vi "L1_selectFile.vi"(7 "Function":T1(ring), 9 "File_Name":string[](array[string]), 11 "dup path":path) -> (1 "FileName":string[](array[string]), 3 "FileName_path":path[](array[path]))   [LabVIEW 2023]
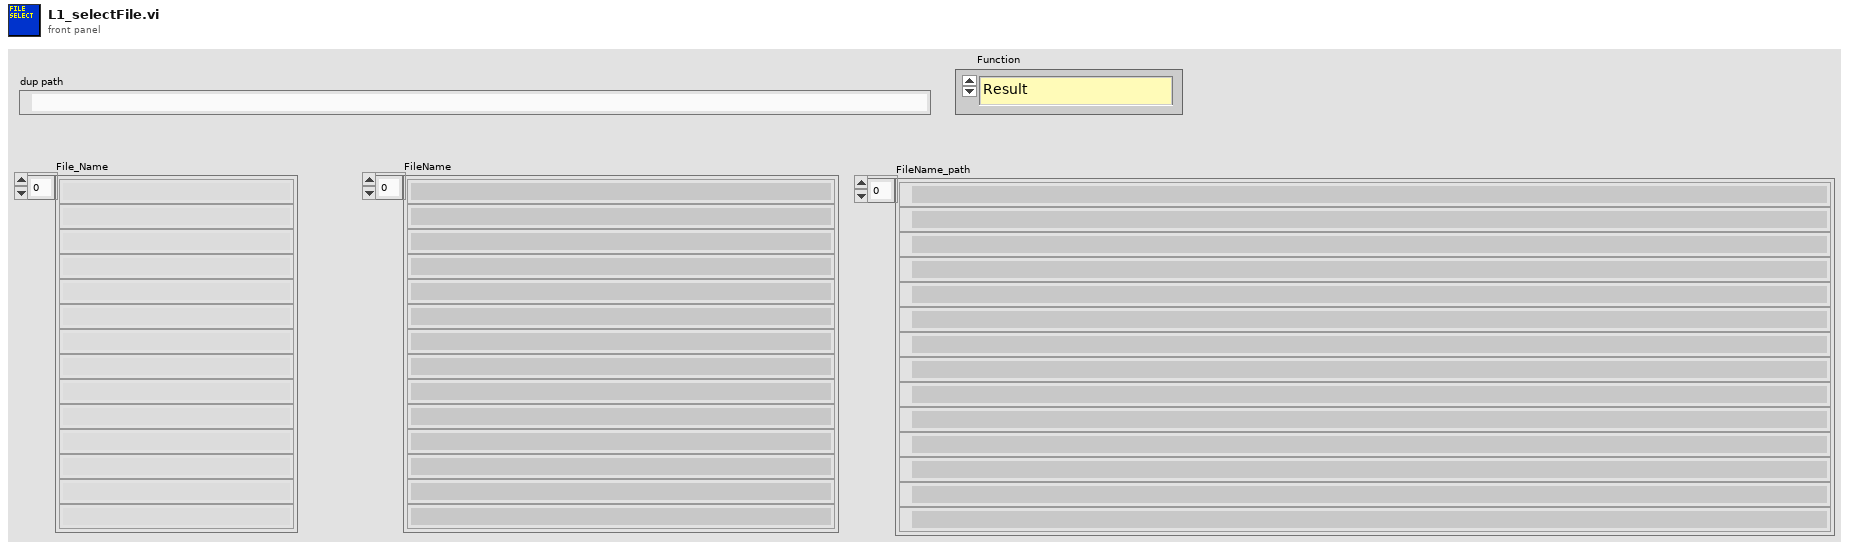
[diagram p1: front panel]
types:
  T1 = enum16{"Result", "Marker_1_26.5GHz", "Marker_2_28GHz", "Marker_3_29.5GHz", "Marker_4_31GHz"}
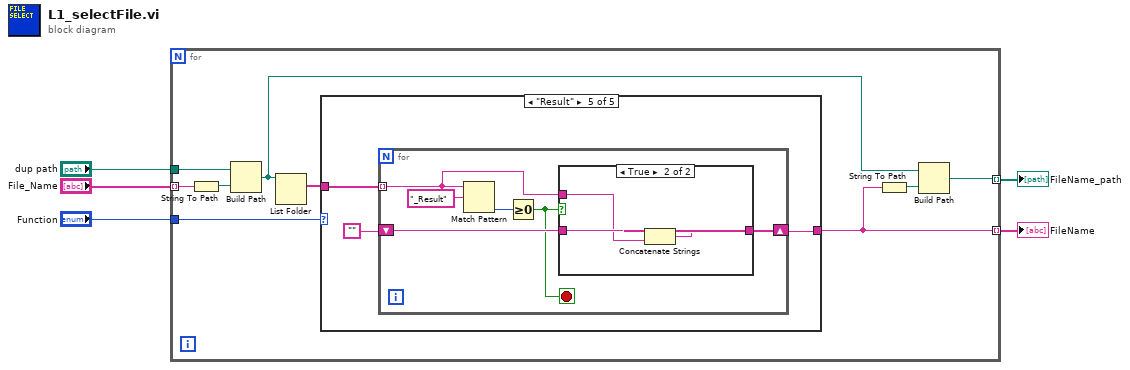
[diagram p0: block diagram]
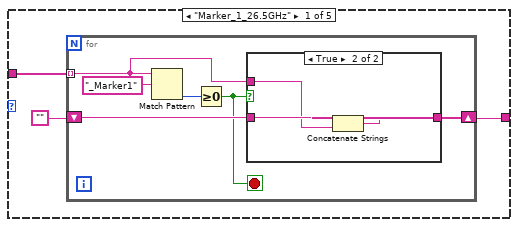
[diagram p2: hidden frame]
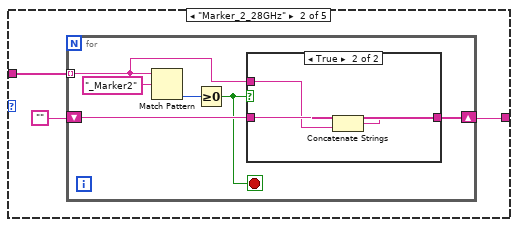
[diagram p4: hidden frame]
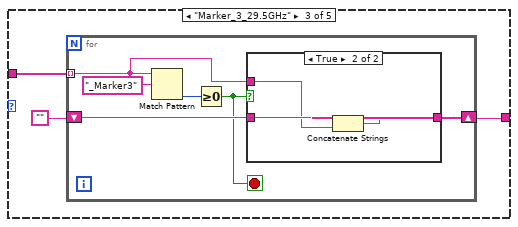
[diagram p6: hidden frame]
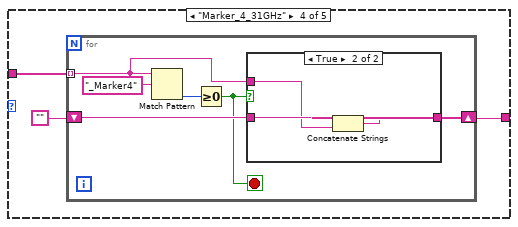
[diagram p8: hidden frame]
diagram:
  n1 = for {
    tunnel: "Function" -> [w14]
    tunnel: "File_Name" -> [w9] mode=indexing
    tunnel: "dup path" -> [w10]
    tunnel: [w12] -> w2 mode=indexing
    tunnel: [w6] -> w1 mode=indexing
    n2 = String To Path(string=w9) -> (path=w11:path)
    n3 = Build Path(base path=w10, name or relative path=w11) -> (appended path=w7:path)
    n4 = List Folder(path=w7) -> (filenames=w8:string[])  [unwired: 3 in, 3 out]
    n5 = case shown="\"Result\"" w14 {
      tunnel: w8 -> [w15 w28 w41 w54 w67]
      tunnel: [w17 w30 w43 w56 w69] -> w12
      frame "Marker_1_26.5GHz" {
        n6 = for {
          tunnel: w15 -> [w21] mode=indexing
          shift-right: [w19] -> w17
          shift-left: "" -> [w20]
          stop <- w18 stop-if-true
          n7 = Match Pattern(string=w21, regular expression="_Marker1") -> (offset past match=w22:i32)  [unwired: 1 in, 3 out]
          n8 = Greater Or Equal To 0?(x=w22) -> (x >= 0?=w18:bool)
          n9 = case shown="True" w18 {
            tunnel: w21 -> [_ w26]
            tunnel: w20 -> [w24 w27]
            tunnel: [w24 w25] -> w19
            frame False {
            }
            frame True {
              n10 = Concatenate Strings(w27, w26) -> (w25:string)
            }
          }
        }
      }
      frame "Marker_2_28GHz" {
        n11 = for {
          tunnel: w28 -> [w34] mode=indexing
          shift-right: [w32] -> w30
          shift-left: "" -> [w33]
          stop <- w31 stop-if-true
          n12 = Match Pattern(string=w34, regular expression="_Marker2") -> (offset past match=w35:i32)  [unwired: 1 in, 3 out]
          n13 = Greater Or Equal To 0?(x=w35) -> (x >= 0?=w31:bool)
          n14 = case shown="True" w31 {
            tunnel: w34 -> [_ w39]
            tunnel: w33 -> [w37 w40]
            tunnel: [w37 w38] -> w32
            frame False {
            }
            frame True {
              n15 = Concatenate Strings(w40, w39) -> (w38:string)
            }
          }
        }
      }
      frame "Marker_3_29.5GHz" {
        n16 = for {
          tunnel: w41 -> [w47] mode=indexing
          shift-right: [w45] -> w43
          shift-left: "" -> [w46]
          stop <- w44 stop-if-true
          n17 = Match Pattern(string=w47, regular expression="_Marker3") -> (offset past match=w48:i32)  [unwired: 1 in, 3 out]
          n18 = Greater Or Equal To 0?(x=w48) -> (x >= 0?=w44:bool)
          n19 = case shown="True" w44 {
            tunnel: w47 -> [_ w52]
            tunnel: w46 -> [w50 w53]
            tunnel: [w50 w51] -> w45
            frame False {
            }
            frame True {
              n20 = Concatenate Strings(w53, w52) -> (w51:string)
            }
          }
        }
      }
      frame "Marker_4_31GHz" {
        n21 = for {
          tunnel: w54 -> [w60] mode=indexing
          shift-right: [w58] -> w56
          shift-left: "" -> [w59]
          stop <- w57 stop-if-true
          n22 = Match Pattern(string=w60, regular expression="_Marker4") -> (offset past match=w61:i32)  [unwired: 1 in, 3 out]
          n23 = Greater Or Equal To 0?(x=w61) -> (x >= 0?=w57:bool)
          n24 = case shown="True" w57 {
            tunnel: w60 -> [_ w65]
            tunnel: w59 -> [w63 w66]
            tunnel: [w63 w64] -> w58
            frame False {
            }
            frame True {
              n25 = Concatenate Strings(w66, w65) -> (w64:string)
            }
          }
        }
      }
      frame "Result" {
        n26 = for {
          tunnel: w67 -> [w73] mode=indexing
          shift-right: [w71] -> w69
          shift-left: "" -> [w72]
          stop <- w70 stop-if-true
          n27 = Match Pattern(string=w73, regular expression="_Result") -> (offset past match=w74:i32)  [unwired: 1 in, 3 out]
          n28 = Greater Or Equal To 0?(x=w74) -> (x >= 0?=w70:bool)
          n29 = case shown="True" w70 {
            tunnel: w73 -> [_ w78]
            tunnel: w72 -> [w76 w79]
            tunnel: [w76 w77] -> w71
            frame False {
            }
            frame True {
              n30 = Concatenate Strings(w79, w78) -> (w77:string)
            }
          }
        }
      }
    }
    n31 = String To Path(string=w12) -> (path=w13:path)
    n32 = Build Path(base path=w7, name or relative path=w13) -> (appended path=w6:path)
  }
  "FileName" <- w2
  "FileName_path" <- w1
